vi "属性节点实例1.vi"() -> ()   [LabVIEW 2023]
panel:
  out "Numeric 2":i32
  in  "stop 2":bool
  in  "Knob":dbl(knob) scale=0.0..100.0
  out "Numeric":i32
  in  "stop":bool
  # "属性节点实例 1"
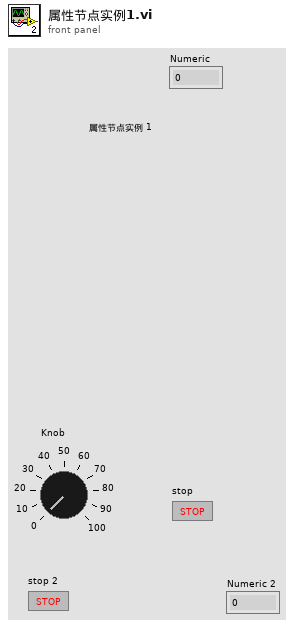
[diagram p1: front panel]
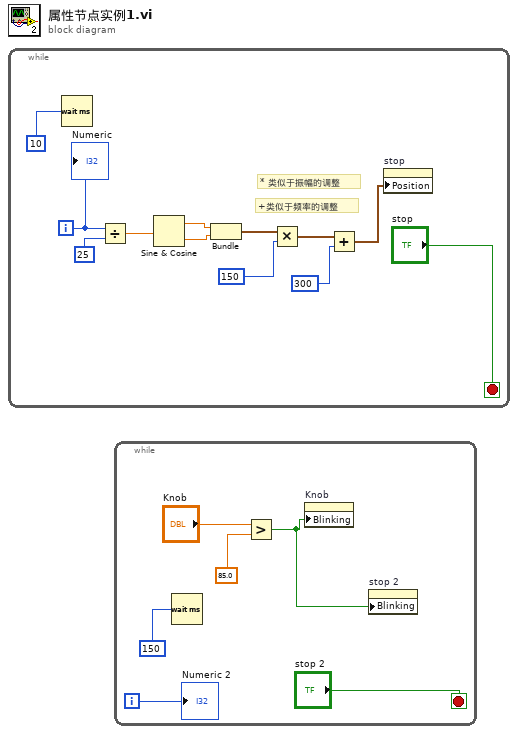
[diagram p0: block diagram]
diagram:
  n1 = while {
    i -> [w1]
    stop <- "stop" stop-if-true
    # "+类似于频率的调整"
    # "* 类似于振幅的调整"
    n2 = Wait (ms)(milliseconds to wait=u32 10) -> ()  [unwired: 1 out]
    n3 = Divide(x=w1, y=25) -> (x/y=w10:dbl)
    n4 = Sine & Cosine(0:w10) -> (1:w9:dbl, 2:w8:dbl)
    n5 = Bundle(w9, w8) -> (w7:cluster{dbl, dbl})  [unwired: 1 in]
    n6 = Multiply(x=w7, y=150) -> (x*y=w6:cluster{dbl, dbl})
    n7 = Add(x=w6, y=300) -> (x+y=w2:cluster{dbl, dbl})
    n8 = property on="stop" class="Bool"("Position"=w2) -> ()  [unwired: 2 in, 2 out]
    "Numeric" <- w1
  }
  n9 = while {
    i -> [w13]
    stop <- "stop 2" stop-if-true
    n10 = Wait (ms)(milliseconds to wait=u32 150) -> ()  [unwired: 1 out]
    n11 = Greater?(x="Knob", y=85.0) -> (0:w15:bool)
    n12 = property on="Knob" class="Knob (strict)"("Blinking"=w15) -> ()  [unwired: 2 in, 2 out]
    n13 = property on="stop 2" class="Bool"("Blinking"=w15) -> ()  [unwired: 2 in, 2 out]
    "Numeric 2" <- w13
  }
